vi "SwerveMath.vi"(5 "Center of Rotation Joystick Axes":cluster{"X":dbl, "Y":dbl}, 6 "Sensor positions":cluster{"FL":dbl, "FR":dbl, "RL":dbl, "RR":dbl}, 7 "Trigger Axes":cluster{"Left":dbl, "Right":dbl}, 9 "Angle (degrees; 0 = right)":dbl, 10 "FieldCentric? (T)":bool=TRUE, 11 "Strafe Joystick Axes":cluster{"X":dbl, "Y":dbl}) -> (1 "Angle Cluster":T1 {"FL Angle" scale=3.1416..-3.1416; "FR Angle" scale=3.1416..-3.1416; "RR Angle" scale=3.1416..-3.1416; "RL Angle" scale=3.1416..-3.1416}, 3 "Speed Cluster":T2 {"RR Speed" scale=-1.0..1.0; "RL Speed" scale=-1.0..1.0; "FR Speed" scale=-1.0..1.0; "FL Speed" scale=-1.0..1.0})   [LabVIEW 2014]
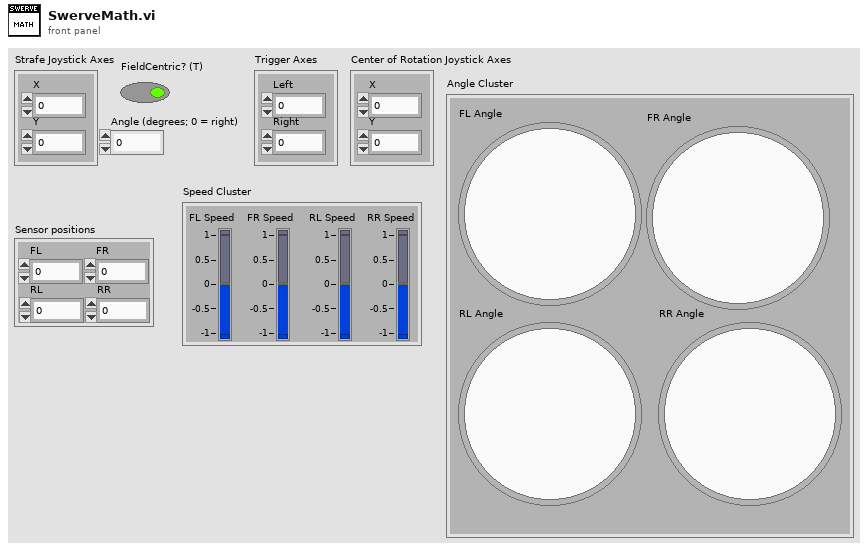
[diagram p1: front panel]
types:
  T1 = cluster{"FL Angle":dbl, "FR Angle":dbl, "RL Angle":dbl, "RR Angle":dbl}
  T2 = cluster{"FL Speed":dbl, "FR Speed":dbl, "RL Speed":dbl, "RR Speed":dbl}
  T3 = cluster{"normalized array[0]":dbl, "normalized array[1]":dbl, "normalized array[2]":dbl, "normalized array[3]":dbl}
  T4 = cluster{"[0]":dbl, "[1]":dbl, "[2]":dbl, "[3]":dbl}
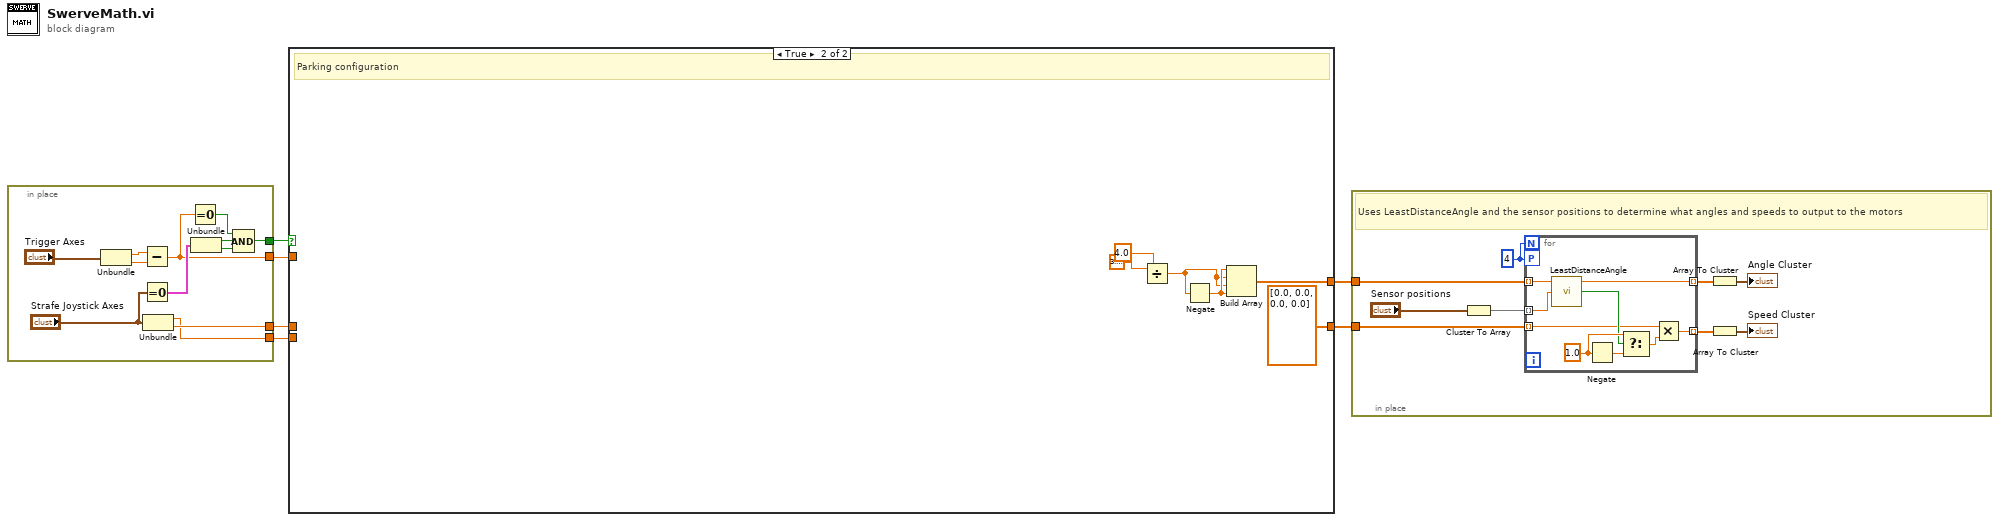
[diagram p0: block diagram]
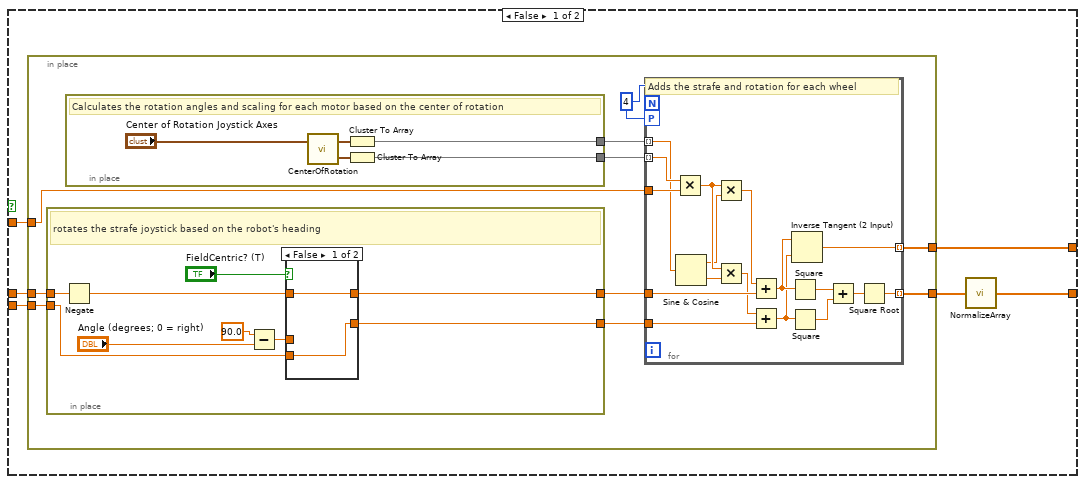
[diagram p2: hidden frame]
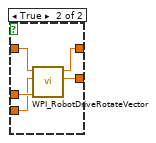
[diagram p3: hidden frame]
diagram:
  n1 = in-place {
    in-place-border: [w10] -> w6
    in-place-border: [w9] -> w3
    in-place-border: [w8] -> w2
    in-place-border: [w7] -> w1
    n2 = Unbundle("Trigger Axes") -> ("Left"=w14:dbl, "Right"=w15:dbl)
    n3 = Subtract(x=w14, y=w15) -> (x-y=w7:dbl)
    n4 = Equal To 0?(x="Strafe Joystick Axes") -> (x = 0?=w17:cluster{"X":bool, "Y":bool})
    n5 = Unbundle("Strafe Joystick Axes") -> ("X"=w8:dbl, "Y"=w9:dbl)
    n6 = Equal To 0?(x=w7) -> (x = 0?=w13:bool)
    n7 = Unbundle(w17) -> ("X"=w12:bool, "Y"=w11:bool)
    n8 = Compound Arithmetic op=AND(w13, w12, w11) -> (w10:bool)
  }
  n9 = case shown="True" w6 {
    tunnel: [w19 w78] -> w5
    tunnel: [w24 dbl[] [0.0, 0.0, 0.0, 0.0] ("appended array")] -> w4
    tunnel: w3 -> [w22 _]
    tunnel: w2 -> [w21 _]
    tunnel: w1 -> [w20 _]
    frame False {
      n10 = in-place {
        in-place-border: [w32] -> w23
        in-place-border: [w31] -> w19
        in-place-border: w22 -> [w29]
        in-place-border: w21 -> [w28]
        in-place-border: w20 -> [w27]
        w30 = 4
        n11 = in-place {
          in-place-border: [w48] -> w34
          in-place-border: [w47] -> w33
          in-place-border: w29 -> [w41]
          in-place-border: w28 -> [w40]
          # "rotates the strafe joystick based on the robot's heading"
          n12 = Negate(x=w41) -> (-x=w42:dbl)
          n13 = Subtract(x=90.0 ("y"), y="Angle (degrees; 0 = right)") -> (x-y=w45:dbl)
          n14 = case shown="False" "FieldCentric? (T)" {
            tunnel: w42 -> [w50 w55]
            tunnel: [w50 w54] -> w48
            tunnel: [w49 w53] -> w47
            tunnel: w45 -> [_ w52]
            tunnel: w40 -> [w49 w51]
            frame False {
            }
            frame True {
              n15 = call <vilib>:"WPI_RobotDriveRotateVector.vi"("Angle"=w52, "X"=w51, "Y"=w55) -> ("X'"=w53:dbl, "Y'"=w54:dbl)  [unwired: 7 out]
            }
          }
        }
        n16 = in-place {
          in-place-border: [w35] -> w26
          in-place-border: [w36] -> w25
          # "Calculates the rotation angles and scaling for each motor based on the center of rotation"
          n17 = call "CenterOfRotation.vi"("Center of Rotation Joystick Axes"="Center of Rotation Joystick Axes") -> ("Rotation Multipliers"=w38:T3, "Rotation Angle Cluster"=w37:T1)  [unwired: 1 in]
          n18 = Cluster To Array(cluster=w37) -> (array=w36:dbl[])
          n19 = Cluster To Array(cluster=w38) -> (array=w35:dbl[])
        }
        n20 = for {
          N: w30 -> [_]
          tunnel: w34 -> [w72]
          tunnel: w33 -> [w71]
          tunnel: w27 -> [w70]
          tunnel: [w69] -> w32 mode=indexing
          tunnel: [w68] -> w31 mode=indexing
          workers-P: w30 -> [_]
          tunnel: w26 -> [w57] mode=indexing
          tunnel: w25 -> [w56] mode=indexing
          # "Adds the strafe and rotation for each wheel"
          n21 = Multiply(x=w57, y=w70) -> (x*y=w60:dbl)
          n22 = Sine & Cosine(0:w56) -> (1:w59:dbl, 2:w58:dbl)
          n23 = Multiply(x=w60, y=w59) -> (x*y=w63:dbl)
          n24 = Multiply(x=w60, y=w58) -> (x*y=w64:dbl)
          n25 = Add(x=w63, y=w72) -> (x+y=w62:dbl)
          n26 = Add(x=w64, y=w71) -> (x+y=w61:dbl)
          n27 = Square(x=w62) -> (x^2=w66:dbl)
          n28 = Square(x=w61) -> (x^2=w65:dbl)
          n29 = Inverse Tangent (2 Input)(1:w61, 2:w62) -> (0:w68:dbl)
          n30 = Add(x=w66, y=w65) -> (x+y=w67:dbl)
          n31 = Square Root(x=w67) -> (sqrt(x)=w69:dbl)
        }
      }
      n32 = call "NormalizeArray.vi"("array"=w23) -> ("normalized array"=w24:dbl[])
    }
    frame True {
      # "Parking configuration"
      n33 = Divide(x=3.141592653589793, y=4.0) -> (x/y=w75:dbl)
      n34 = Negate(x=w75) -> (-x=w76:dbl)
      n35 = Build Array(w76, w75, w75, w76) -> (w78:dbl[])
    }
  }
  n36 = in-place {
    in-place-border: w5 -> [w87]
    in-place-border: w4 -> [w85]
    w79 = 4
    # "Uses LeastDistanceAngle and the sensor positions to determine what angles and speeds to output to the motors"
    n37 = Cluster To Array(cluster="Sensor positions") -> (array=w86:dbl[])
    n38 = for {
      N: w79 -> [_]
      workers-P: w79 -> [_]
      tunnel: w87 -> [w96] mode=indexing
      tunnel: w86 -> [w95] mode=indexing
      tunnel: [w90] -> w83 mode=indexing
      tunnel: w85 -> [w89] mode=indexing
      tunnel: [w88] -> w84 mode=indexing
      w94 = 1.0 ("t")
      n39 = call "LeastDistanceAngle.vi"("Sensor position"=w95, "target angle (between pi and -pi)"=w96) -> ("Reverse?"=w92:bool, "motor output angle"=w88:dbl)  [unwired: 1 in, 1 out]
      n40 = Negate(x=w94) -> (-x=w93:dbl)
      n41 = Select(t=w94, s=w92, f=w93) -> (s? t:f=w91:dbl)
      n42 = Multiply(x=w89, y=w91) -> (x*y=w90:dbl)
    }
    n43 = Array To Cluster(array=w84) -> (cluster=→"Angle Cluster":T4)
    n44 = Array To Cluster(array=w83) -> (cluster=→"Speed Cluster":T4)
  }
